vi "Get Position.vi"(8 "error in (no error)":errorcluster, 10 "Axis":i32=1, 11 "Simulated in":refnum<class "Simulated-TS.lvclass">) -> (0 "error out":errorcluster, 1 "Position":dbl, 3 "Simulated out":refnum<class "Simulated-TS.lvclass">)   [LabVIEW 2019, in "Simulated-TS.lvclass"]
uses:
  Simulated-TS.lvclass
  Simulated-TS.lvclass/Simulated-TS.ctl
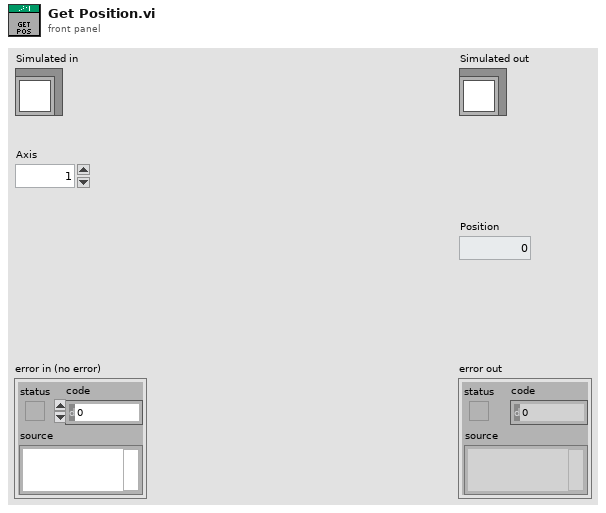
[diagram p1: front panel]
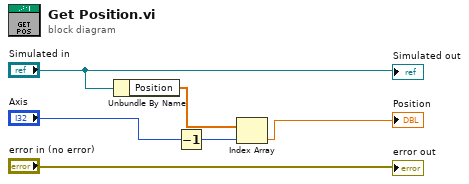
[diagram p0: block diagram]
diagram:
  n1 = Unbundle By Name("Simulated in") -> ("Position"=w5:dbl[])
  n2 = Decrement(x="Axis") -> (x-1=w3:i32)
  n3 = Index Array(array=w5, index=w3) -> (element=→"Position":dbl)
  "error out" <- "error in (no error)"
  "Simulated out" <- "Simulated in"
